vi "1 PulseMeasurement.vi"(2 "PulseMeas Ch":refnum<k21>="Connector0/DIO0", 4 "PulseMeas 0 Timeout":u32=40000) -> (7 "PulseMeas Packet":u64)   [LabVIEW 2010]
uses:
  <vilib>/eio/EIONode/EIONode.xnode
  <vilib>/NI Veristand/FPGA/NI_VS FPGA Support.lvlib
  <vilib>/rvi/eio/nirviEIOImplementation/nirviEIOImplementation.xnode
  <vilib>/rvi/eio/common/nirviEmuTemplateMethod_noerrors.vi
  <vilib>/rvi/eio/common/nirviEmuClasses.ctl
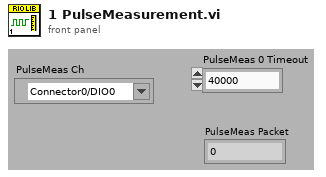
[diagram p1: front panel]
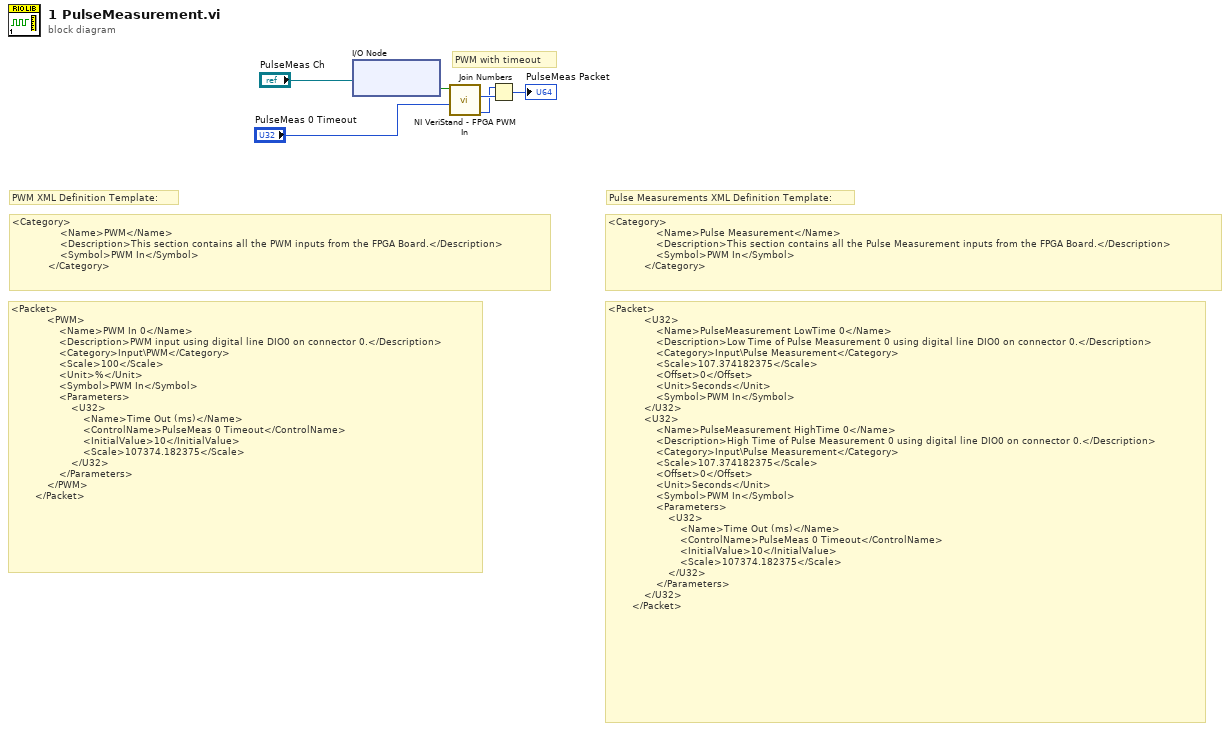
[diagram p0: block diagram]
diagram:
  # "<Category>\n                <Name>PWM</Name>\n                <Description>This section contains all the PWM inputs from the FPGA Board.</Description>\n                <Symbol>PWM In</Symbol>\n            </Category>"
  # "<Category>\n                <Name>Pulse Measurement</Name>\n                <Description>This section contains all the Pulse Measurement inputs from the FPGA Board.</Description>\n                <Symbol>PWM In</Symbol>\n            </Category>"
  # "Pulse Measurements XML Definition Template:"
  # "PWM XML Definition Template:"
  # "<Packet>\n            <PWM>\n                <Name>PWM In 0</Name>\n                <Description>PWM input using digital line DIO0 on connector 0.</Description>\n                <Category>Input\\PWM</Category>\n                <Scale>100</Scale>\n                <Unit>%</Unit>\n                <Symbol>PWM In</Symbol>\n                <Parameters>\n                    <U32>\n                        <Name>Time Out (ms)</Name>\n                        <ControlName>PulseMeas 0 Timeout</ControlName>\n                        <InitialValue>10</InitialValue>\n                        <Scale>107374.182375</Scale>\n                    </U32>\n                </Parameters>\n            </PWM>\n        </Packet>"
  # "<Packet>\n            <U32>\n                <Name>PulseMeasurement LowTime 0</Name>\n                <Description>Low Time of Pulse Measurement 0 using digital line DIO0 on connector 0.</Description>\n                <Category>Input\\Pulse Measurement</Category>\n                <Scale>107.374182375</Scale>\n                <Offset>0</Offset>\n                <Unit>Seconds</Unit>\n                <Symbol>PWM In</Symbol>\n            </U32>\n            <U32>\n                <Name>PulseMeasurement HighTime 0</Name>\n                <Description>High Time of Pulse Measurement 0 using digital line DIO0 on connector 0.</Description>\n                <Category>Input\\Pulse Measurement</Category>\n                <Scale>107.374182375</Scale>\n                <Offset>0</Offset>\n                <Unit>Seconds</Unit>\n                <Symbol>PWM In</Symbol>\n                <Parameters>\n                    <U32>\n                        <Name>Time Out (ms)</Name>\n                        <ControlName>PulseMeas 0 Timeout</ControlName>\n                        <InitialValue>10</InitialValue>\n                        <Scale>107374.182375</Scale>\n                    </U32>\n                </Parameters>\n            </U32>\n        </Packet>"
  # "PWM with timeout"
  n1 = xnode "I/O Node"("FPGA I/O In"="PulseMeas Ch") -> ("I/O Item"=w6:bool)  [unwired: 1 out]
  n2 = call <vilib>:"NI VeriStand - FPGA PWM In.vi"("Time Out"="PulseMeas 0 Timeout", "Value"=w6) -> ("High time"=w2:u32, "Low Time"=w3:u32)  [unwired: 8 out]
  n3 = Join Numbers(hi=w2, lo=w3) -> ((hi.lo)=→"PulseMeas Packet":u64)
